vi "Kikusui PLZ-Configure Response Speed.vi"(8 "error in":errorcluster, 10 "Response Speed":u16(ring) items=["Normal Response Speed", "1/2 the Normal Response Speed", "1/5 the Normal Response Speed", "1/10 the Normal Response Speed"], 11 "Kikusui PLZ Setting In":T1={"VISA Resource Name"="", "Baud Rate"=19200, "Stop Bits"=20, "Wait For Read(ms)"=0} {"Stop Bits" items=["1.0"=10, "2.0"=20]; "Baud Rate" items=["2400"=2400, "4800"=4800, "9600"=9600, "19200"=19200]}) -> (0 "error out":errorcluster, 3 "Kikusui PLZ Setting Out":T1={"VISA Resource Name"="", "Baud Rate"=19200, "Stop Bits"=20, "Wait For Read(ms)"=0} {"Stop Bits" items=["1.0"=10, "2.0"=20]; "Baud Rate" items=["2400"=2400, "4800"=4800, "9600"=9600, "19200"=19200]})   [LabVIEW 2018]
doc: "Configures the response speed of the instrument. The PLZ4W operates by detecting the input current or voltage and feeding back those values. You can decrease the response speed to assure stable operation.\n\n<b>Note:</b>\n1) Works in CC,CR, CC+CV and CR+CV mode."
uses:
  Data Def/Kikusui PLZ-Setting.ctl
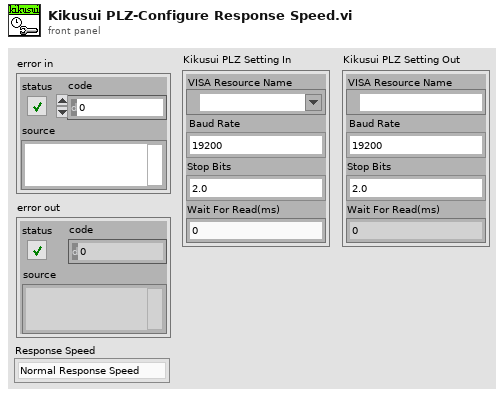
[diagram p1: front panel]
types:
  T1 = typedef "Kikusui PLZ-Setting.ctl" = cluster{"VISA Resource Name":refnum<visa-resource-name>, "Baud Rate":u32, "Stop Bits":u16, "Wait For Read(ms)":u32}
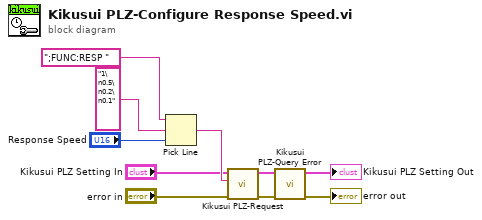
[diagram p0: block diagram]
diagram:
  n1 = Pick Line(string ("")=";FUNC:RESP ", multi-line string="1\n0.5\n0.2\n0.1", line index="Response Speed") -> (output string=w3:string)
  n2 = call "Kikusui PLZ-Request.vi"("error in"="error in", "Command"=w3, "Kikusui PLZ Setting In"="Kikusui PLZ Setting In") -> ("error out"=w6:errorcluster, "Kikusui PLZ Setting Out"=w5:T1)  [unwired: 6 in, 1 out]
  n3 = call "Kikusui PLZ-Query Error.vi"("error in"=w6, "Kikusui PLZ Setting In"=w5) -> ("error out"=→"error out":errorcluster, "Kikusui PLZ Setting Out"=→"Kikusui PLZ Setting Out":T1)  [unwired: 8 in]
